vi "FlowCalculations.vi"(0 "FlowGPH":dbl, 1 "Temp Coe":dbl, 5 "SGH20":dbl, 7 "Fuel Temp":dbl, 9 "SGi":dbl, 11 "error in (no error)":errorcluster, 12 "Ti":dbl) -> (4 "Flow Lb/hr":dbl, 6 "SGCal":dbl, 15 "error out":errorcluster)   [LabVIEW 2018]
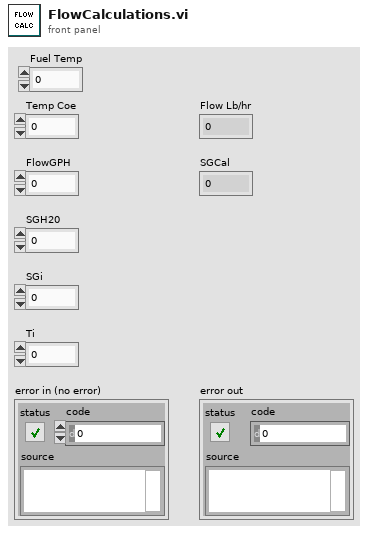
[diagram p1: front panel]
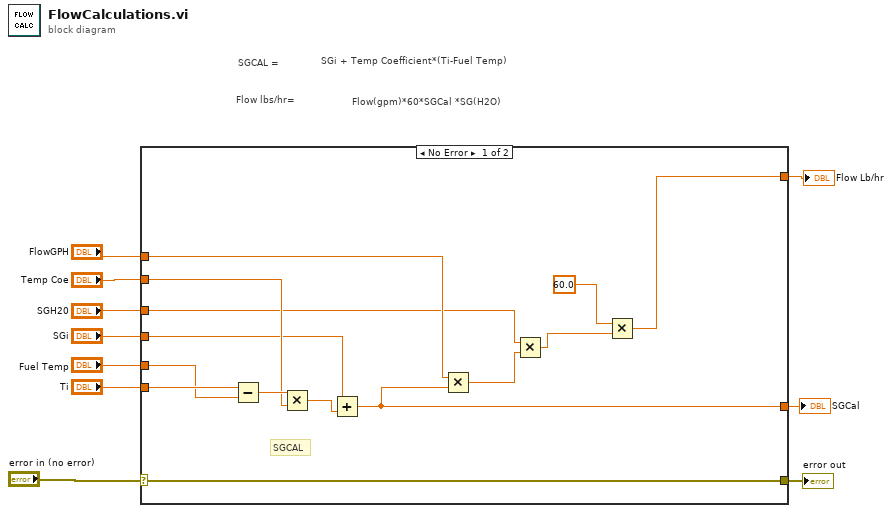
[diagram p0: block diagram]
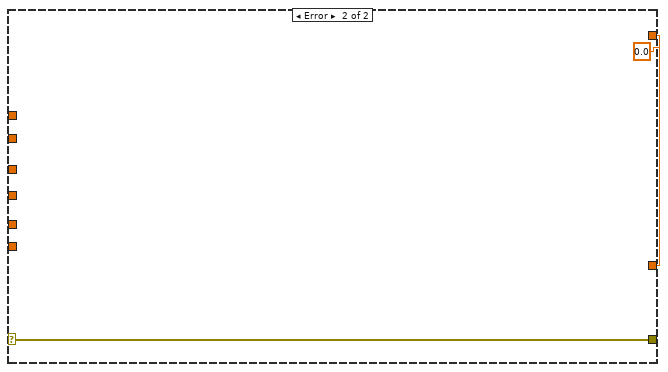
[diagram p2: hidden frame]
diagram:
  # "Flow lbs/hr="
  # "SGi + Temp Coefficient*(Ti-Fuel Temp)"
  # "Flow(gpm)*60*SGCal *SG(H2O)"
  # "SGCAL ="
  n1 = case shown="No Error" "error in (no error)" {
    selector: "error in (no error)" -> [w24 w25]
    tunnel: [w24 w25] -> w3
    tunnel: [w13 w26] -> w9
    tunnel: [w19 w26] -> w10
    tunnel: "FlowGPH" -> [w18 _]
    tunnel: "Temp Coe" -> [w20 _]
    tunnel: "SGH20" -> [w16 _]
    tunnel: "SGi" -> [w11 _]
    tunnel: "Ti" -> [w23 _]
    tunnel: "Fuel Temp" -> [w22 _]
    frame No Error {
      # "SGCAL"
      n2 = Subtract(x=w23, y=w22) -> (x-y=w21:dbl)
      n3 = Multiply(x=w21, y=w20) -> (x*y=w12:dbl)
      n4 = Add(x=w11, y=w12) -> (x+y=w19:dbl)
      n5 = Multiply(x=w18, y=w19) -> (x*y=w17:dbl)
      n6 = Multiply(x=w16, y=w17) -> (x*y=w15:dbl)
      n7 = Multiply(x=60.0, y=w15) -> (x*y=w13:dbl)
    }
    frame Error {
      w26 = 0.0
    }
  }
  "SGCal" <- w10
  "Flow Lb/hr" <- w9
  "error out" <- w3
